vi "Initialize.vi"(8 "error in (no error)":errorcluster, 10 "DeviceName":string, 11 "FakePressureController in":refnum<class "MagAnalysis_Online.lvclass">) -> (0 "error out":errorcluster, 1 "new command(s)":string, 2 "DeviceName":string, 3 "FakePressureController out":refnum<class "MagAnalysis_Online.lvclass">)   [LabVIEW 2013, in "MagAnalysis_Online.lvclass"]
uses:
  MagAnalysis_Online.lvclass
  settings_TypDef.ctl
  CamSettings_Typdef.ctl
  CamSettingSUB_TypDEf.ctl
  MagAnalysis_Online_Bella/SubVis/CamAndObj_TypDEf.ctl
  shared/OnOffTypeDef.ctl
  SubVis/userROI.ctl
  shared/numericVariable_TypeDef.ctl
  SubVis/CamRoiTypDef.ctl
  SrewMaster_TYpDef.ctl
  srew_TypDEf.ctl
  ScrewSub_Typdef.ctl
  SubVis/screwstart.ctl
  calib_Sub_Typdef.ctl
  SubVis/ScreenCam2_TypDEf.ctl
  SubVis/ROIInfo_TypDef.ctl
  SubVis/calibPixel.ctl
  SubVis/2DTypDef.ctl
  SubVis/finalCalibTypdef.ctl
  SubVis/deltaE_FGV_typdef.ctl
  <vilib>/userdefined/High Color/IMAQdx.ctl
  BaseDriver/BaseDriver.lvclass
  MagAnalysis_Online.lvclass/MagAnalysis_Online.ctl
  SubVis/classicROI_typDef.ctl
  shared/CompressAndUpdate(Poly)/CompressAndUpdate(Numeric).vi
  <vilib>/vision/driver/NI_Vision_Acquisition_Software.lvlib
  <resource>/objmgr/imaqdx.rc
panel:
  out "Clibration.cam 0":T1={"incident ANGLE COMPENSATION"=[], "dp/B [MeV/C/B]"=[], "charge compensation"=[], "Momentum [MeV/C]"=[], "energyDependence Input"=[], "pixel angle (y)"=[], "dp [MeV/C/] "=[], "angle 2Dfor spectrumj"=[], "dp [MeV/C] 2D"=[], "charge compensation 2D"=[], "Screen&Camera 2"={"Screen Orientation"="Regular", "Screen angle"="Flat", "Lens"=enum."FL1-f8x08", "Calibration (mm/pix)"=1.0}, "ROI info"={"npix-X"=0, "npix-Y"=0, "Left [pix]"=0.0, "Top [pix]"=0.0}, "Y 2D full angle"=[], "calib pixel"={"y1(pixel)"=[], "y2(pixel)"=[], "dp/B [MeV/C/B] (pixel)"=[], "energyDependence Input(pixel)"=[], "bending angle [deg](pixel)"=[], "total path(pixel)"=[], "pixel angle (y)(pixel)"=[], "energy dependence (pixel)"=[], "charge compensation (pixel)"=[], "Momentum [MeV/C](pixel)"=[], "angular compensation(pixel)"=[]}, "2D"={"dp"=[], "chargeCompensation"=[], "angle"=[], "Momentum"=[]}, "UserROI"={"Width"=0.0, "Hight"=0.0, "OffsetX"=0.0, "OffsetY"=0.0}, "final"={"X"=[], "xi"=[], "delta momentum"=0.0, "Y"=[], "yi"=[], "angle (Y)"=[], "delta angle"=0.0, "scale delta angle"=0.0, "intraX"=0.0, "intraY"=0.0, "mask"=[]}, "B[T]"=0.0, "index"=0.0}
  out "ROI":i32[][](array[numeric])
  out "data":T9={"CamSettings"={"Cam 0"={"position"=0.0, "pixelsize"=0.0, "start"=0.0, "end"=0.0, "center"=0.0, "Lens"=enum."FL1-f8x08", "Forward"=enum."off", "Spec_Calib_file 2"=path "Y:/100TWdata/ESMCalib/datFwd.txt", "map"=path "Y:/100TWdata/ESMCalib/mapFwd.txt", "y size"=0, "UserROI"={"Width"={"Value"=0.0, "Min"=0.0, "Max"=0.0, "StepSize"=0.0, "Tolerance"=0.0, "ValueActual"=0.0}, "Hight"={"Value"=0.0, "Min"=0.0, "Max"=0.0, "StepSize"=0.0, "Tolerance"=0.0, "ValueActual"=0.0}, "OffsetX"={"Value"=0.0, "Min"=0.0, "Max"=0.0, "StepSize"=0.0, "Tolerance"=0.0, "ValueActual"=0.0}, "OffsetY"={"Value"=0.0, "Min"=0.0, "Max"=0.0, "StepSize"=0.0, "Tolerance"=0.0, "ValueActual"=0.0}}, "CamMaxPixel"={"X"=0, "Y"=0}, "CamROI"={"Width"=0.0, "Hight"=0.0, "OffsetX"=0.0, "OffsetY"=0.0}}, "Cam 1"={"position"=0.0, "pixelsize"=0.0, "start"=0.0, "end"=0.0, "center"=0.0, "Lens"=enum."FL1-f8x08", "Forward"=enum."off", "Spec_Calib_file 2"=path "Y:/100TWdata/ESMCalib/datFwd.txt", "map"=path "Y:/100TWdata/ESMCalib/mapFwd.txt", "y size"=0, "UserROI"={"Width"={"Value"=0.0, "Min"=0.0, "Max"=0.0, "StepSize"=0.0, "Tolerance"=0.0, "ValueActual"=0.0}, "Hight"={"Value"=0.0, "Min"=0.0, "Max"=0.0, "StepSize"=0.0, "Tolerance"=0.0, "ValueActual"=0.0}, "OffsetX"={"Value"=0.0, "Min"=0.0, "Max"=0.0, "StepSize"=0.0, "Tolerance"=0.0, "ValueActual"=0.0}, "OffsetY"={"Value"=0.0, "Min"=0.0, "Max"=0.0, "StepSize"=0.0, "Tolerance"=0.0, "ValueActual"=0.0}}, "CamMaxPixel"={"X"=0, "Y"=0}, "CamROI"={"Width"=0.0, "Hight"=0.0, "OffsetX"=0.0, "OffsetY"=0.0}}, "Cam 2"={"position"=0.0, "pixelsize"=0.0, "start"=0.0, "end"=0.0, "center"=0.0, "Lens"=enum."FL1-f8x08", "Forward"=enum."off", "Spec_Calib_file 2"=path "Y:/100TWdata/ESMCalib/datFwd.txt", "map"=path "Y:/100TWdata/ESMCalib/mapFwd.txt", "y size"=0, "UserROI"={"Width"={"Value"=0.0, "Min"=0.0, "Max"=0.0, "StepSize"=0.0, "Tolerance"=0.0, "ValueActual"=0.0}, "Hight"={"Value"=0.0, "Min"=0.0, "Max"=0.0, "StepSize"=0.0, "Tolerance"=0.0, "ValueActual"=0.0}, "OffsetX"={"Value"=0.0, "Min"=0.0, "Max"=0.0, "StepSize"=0.0, "Tolerance"=0.0, "ValueActual"=0.0}, "OffsetY"={"Value"=0.0, "Min"=0.0, "Max"=0.0, "StepSize"=0.0, "Tolerance"=0.0, "ValueActual"=0.0}}, "CamMaxPixel"={"X"=0, "Y"=0}, "CamROI"={"Width"=0.0, "Hight"=0.0, "OffsetX"=0.0, "OffsetY"=0.0}}, "Cam 3"={"position"=0.0, "pixelsize"=0.0, "start"=0.0, "end"=0.0, "center"=0.0, "Lens"=enum."FL1-f8x08", "Forward"=enum."off", "Spec_Calib_file 2"=path "Y:/100TWdata/ESMCalib/datFwd.txt", "map"=path "Y:/100TWdata/ESMCalib/mapFwd.txt", "y size"=0, "UserROI"={"Width"={"Value"=0.0, "Min"=0.0, "Max"=0.0, "StepSize"=0.0, "Tolerance"=0.0, "ValueActual"=0.0}, "Hight"={"Value"=0.0, "Min"=0.0, "Max"=0.0, "StepSize"=0.0, "Tolerance"=0.0, "ValueActual"=0.0}, "OffsetX"={"Value"=0.0, "Min"=0.0, "Max"=0.0, "StepSize"=0.0, "Tolerance"=0.0, "ValueActual"=0.0}, "OffsetY"={"Value"=0.0, "Min"=0.0, "Max"=0.0, "StepSize"=0.0, "Tolerance"=0.0, "ValueActual"=0.0}}, "CamMaxPixel"={"X"=0, "Y"=0}, "CamROI"={"Width"=0.0, "Hight"=0.0, "OffsetX"=0.0, "OffsetY"=0.0}}}, "timeout"={"Value"=0.0, "Min"=0.0, "Max"=0.0, "StepSize"=0.0, "Tolerance"=0.0, "ValueActual"=0.0}, "Screws"={"Cam 0"={"S 0"={"0"=0, "1"=0, "2"=0, "3"=0}, "S 1"={"0"=0, "1"=0, "2"=0, "3"=0}, "S 2"={"0"=0, "1"=0, "2"=0, "3"=0}, "S 3"={"0"=0, "1"=0, "2"=0, "3"=0}, "S 4"={"0"=0, "1"=0, "2"=0, "3"=0}, "S 5"={"0"=0, "1"=0, "2"=0, "3"=0}}, "Cam 1"={"S 0"={"0"=0, "1"=0, "2"=0, "3"=0}, "S 1"={"0"=0, "1"=0, "2"=0, "3"=0}, "S 2"={"0"=0, "1"=0, "2"=0, "3"=0}, "S 3"={"0"=0, "1"=0, "2"=0, "3"=0}, "S 4"={"0"=0, "1"=0, "2"=0, "3"=0}, "S 5"={"0"=0, "1"=0, "2"=0, "3"=0}}, "Cam 2"={"S 0"={"0"=0, "1"=0, "2"=0, "3"=0}, "S 1"={"0"=0, "1"=0, "2"=0, "3"=0}, "S 2"={"0"=0, "1"=0, "2"=0, "3"=0}, "S 3"={"0"=0, "1"=0, "2"=0, "3"=0}, "S 4"={"0"=0, "1"=0, "2"=0, "3"=0}, "S 5"={"0"=0, "1"=0, "2"=0, "3"=0}}, "Cam 3"={"S 0"={"0"=0, "1"=0, "2"=0, "3"=0}, "S 1"={"0"=0, "1"=0, "2"=0, "3"=0}, "S 2"={"0"=0, "1"=0, "2"=0, "3"=0}, "S 3"={"0"=0, "1"=0, "2"=0, "3"=0}, "S 4"={"0"=0, "1"=0, "2"=0, "3"=0}, "S 5"={"0"=0, "1"=0, "2"=0, "3"=0}}}, "number of cam"=0.0, "X size"=0.0, "srewstart"={"Cam 0"=0.0, "Cam 1"=0.0, "Cam 2"=0.0, "Cam 3"=0.0}, "Save"=enum."off", "offset"=0.0, "localsavingpath"=path "", "ROIString"="", "exposure"={"Value"=0.0, "Min"=0.0, "Max"=0.0, "StepSize"=0.0, "Tolerance"=0.0, "ValueActual"=0.0}, "trigger"=enum."off"}
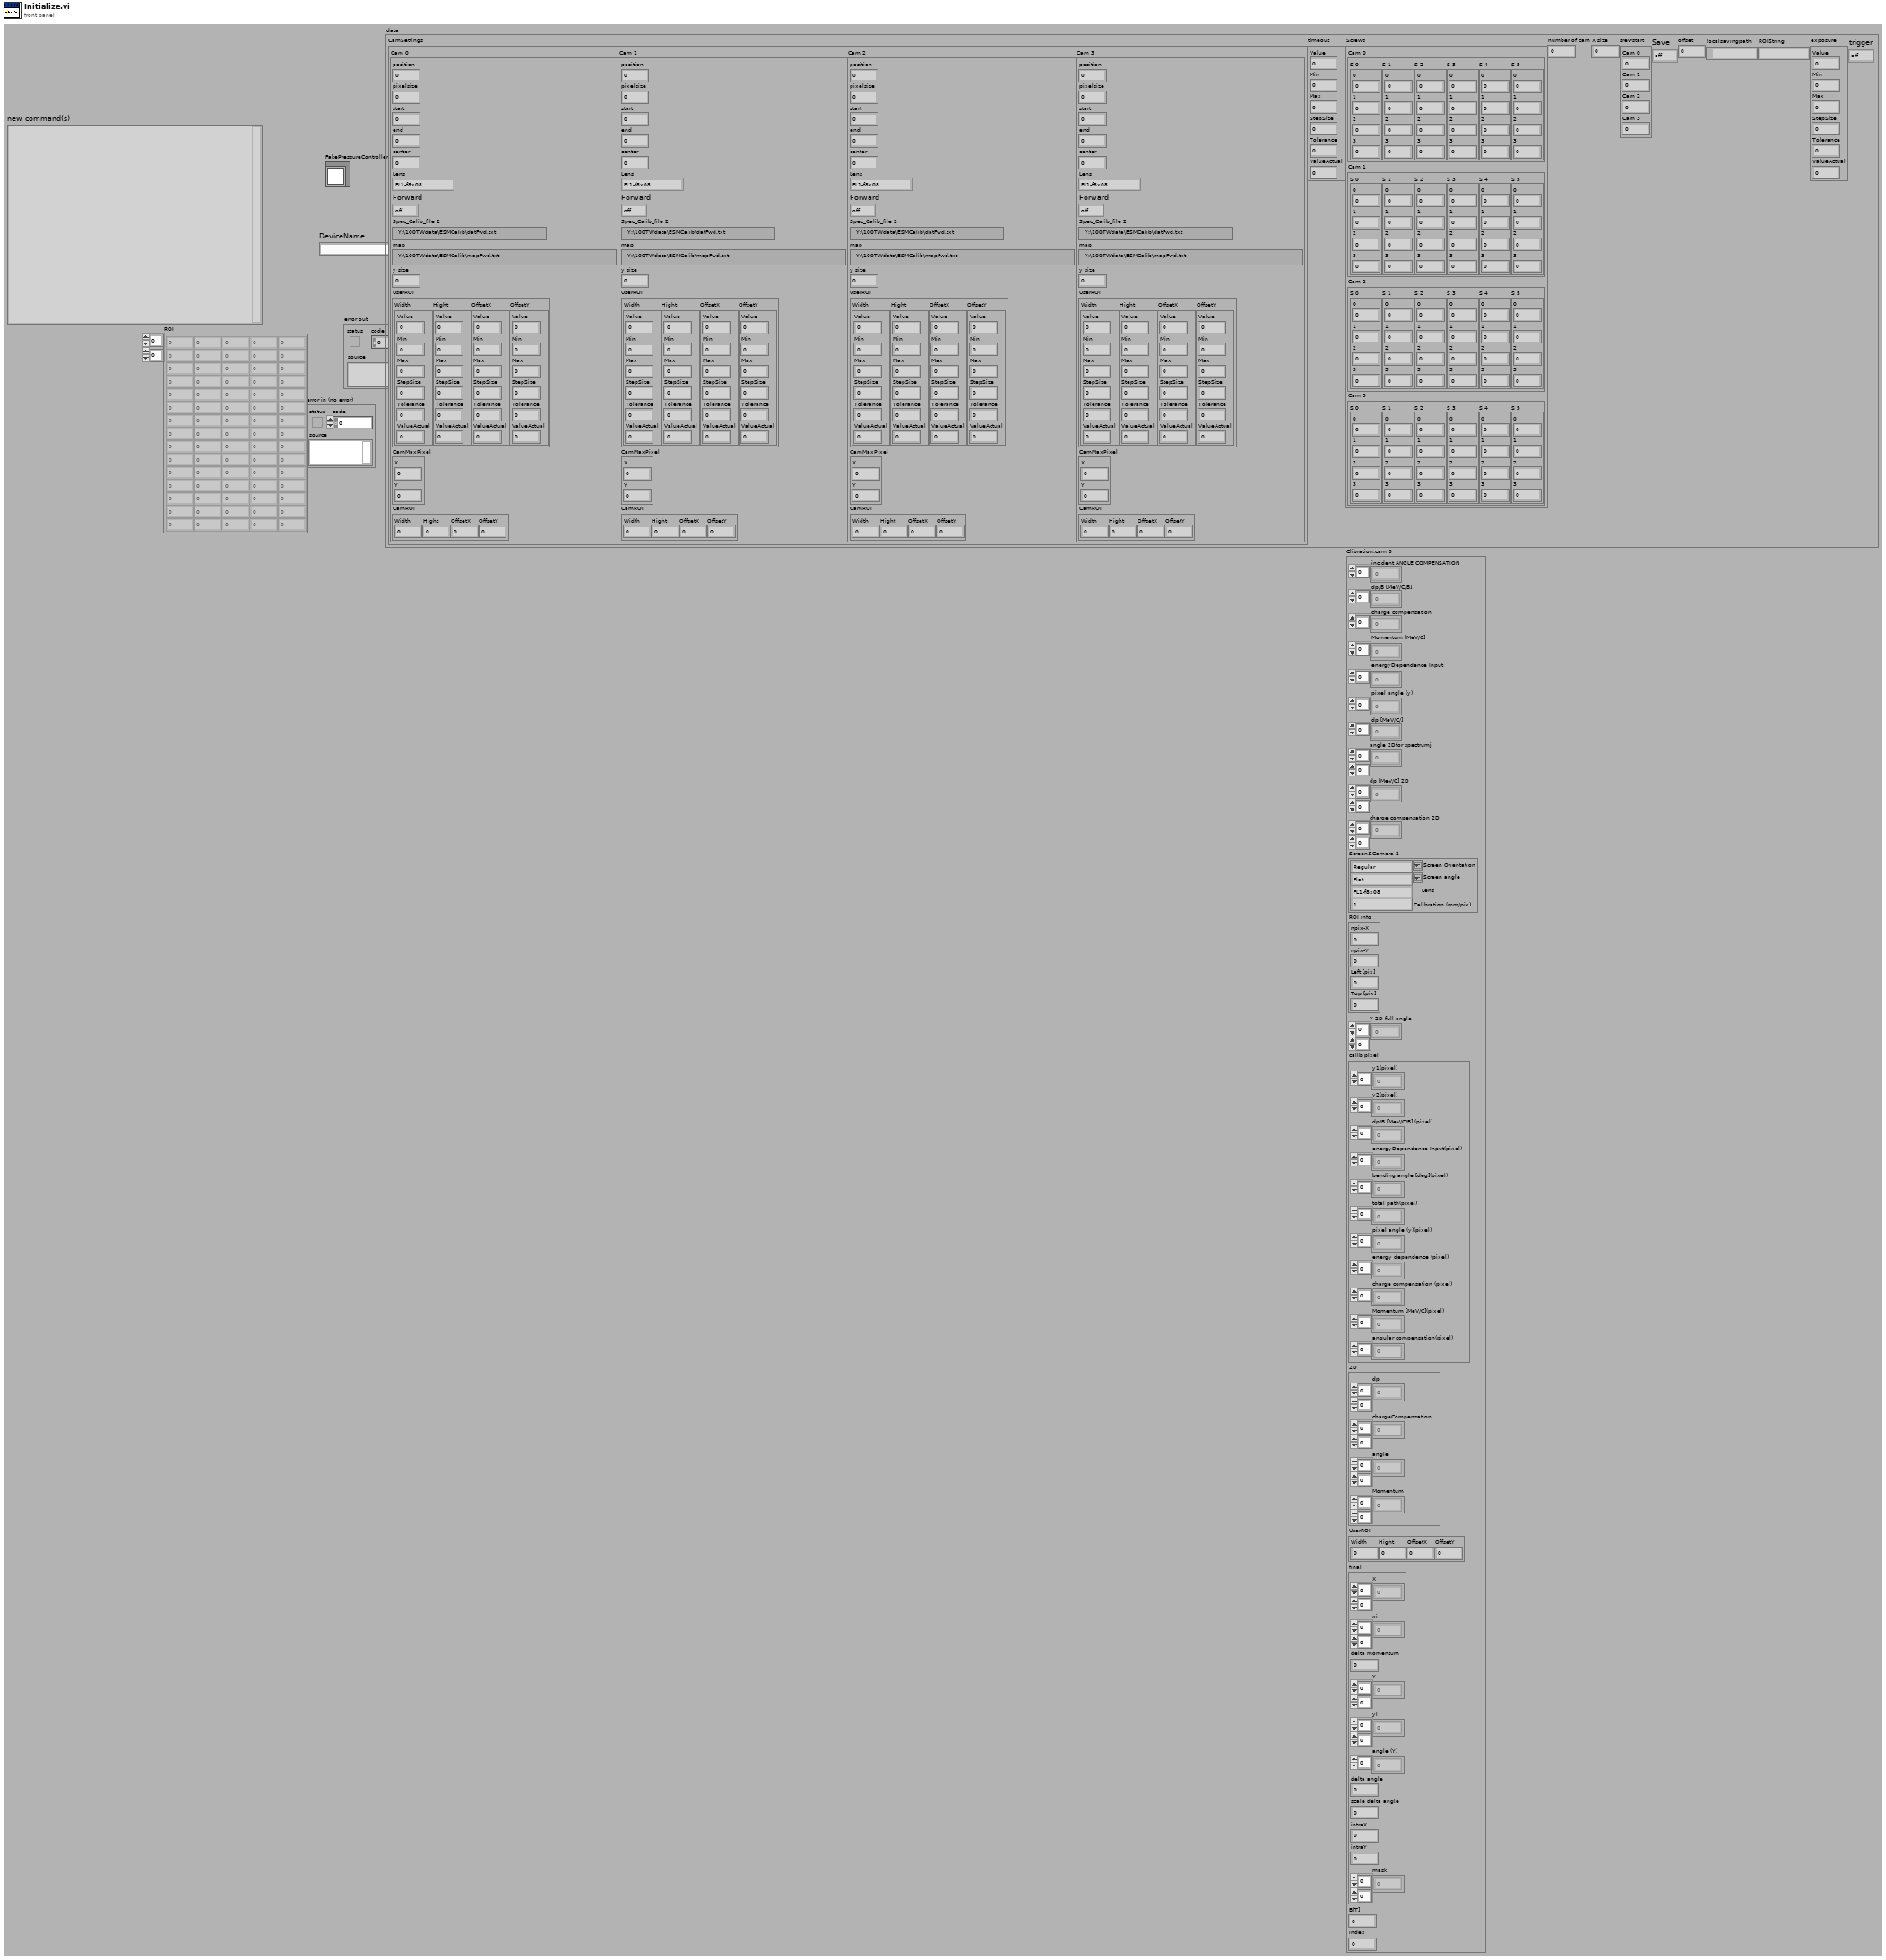
[diagram p1: front panel]
types:
  T1 = typedef "calib_Sub_Typdef.ctl" = cluster{"incident ANGLE COMPENSATION":dbl[], "dp/B [MeV/C/B]":dbl[], "charge compensation":dbl[], "Momentum [MeV/C]":dbl[], "energyDependence Input":dbl[], "pixel angle (y)":dbl[], "dp [MeV/C/] ":dbl[], "angle 2Dfor spectrumj":dbl[][], "dp [MeV/C] 2D":dbl[][], "charge compensation 2D":dbl[][], "Screen&Camera 2":T2, "ROI info":T4, "Y 2D full angle":dbl[][], "calib pixel":T5, "2D":T6, "UserROI":T7, "final":T8, "B[T]":dbl, "index":dbl}
  T2 = typedef "ScreenCam2_TypDEf.ctl" = cluster{"Screen Orientation":string, "Screen angle":string, "Lens":T3, "Calibration (mm/pix)":dbl}
  T3 = typedef "CamAndObj_TypDEf.ctl" = enum16{"FL1-f8x08", "FL1-f8x06", "FL1-f8", "ch300-f50", "FL2G-f8", "FL3M14-f8", "FL3M14-f8x08", "FL3M14-f8x08(2x2)"}
  T4 = typedef "ROIInfo_TypDef.ctl" = cluster{"npix-X":i32, "npix-Y":i32, "Left [pix]":dbl, "Top [pix]":dbl}
  T5 = typedef "calibPixel.ctl" = cluster{"y1(pixel)":dbl[], "y2(pixel)":dbl[], "dp/B [MeV/C/B] (pixel)":dbl[], "energyDependence Input(pixel)":dbl[], "bending angle [deg](pixel)":dbl[], "total path(pixel)":dbl[], "pixel angle (y)(pixel)":dbl[], "energy dependence (pixel)":dbl[], "charge compensation (pixel)":dbl[], "Momentum [MeV/C](pixel)":dbl[], "angular compensation(pixel)":dbl[]}
  T6 = typedef "2DTypDef.ctl" = cluster{"dp":dbl[][], "chargeCompensation":dbl[][], "angle":dbl[][], "Momentum":dbl[][]}
  T7 = typedef "CamRoiTypDef.ctl" = cluster{"Width":dbl, "Hight":dbl, "OffsetX":dbl, "OffsetY":dbl}
  T8 = typedef "finalCalibTypdef.ctl" = cluster{"X":dbl[][], "xi":dbl[][], "delta momentum":dbl, "Y":dbl[][], "yi":dbl[][], "angle (Y)":dbl[], "delta angle":dbl, "scale delta angle":dbl, "intraX":dbl, "intraY":dbl, "mask":dbl[][]}
  T9 = typedef "MagAnalysis_Online.lvclass/settings_TypDef.ctl" = cluster{"CamSettings":T10, "timeout":T14, "Screws":T15, "number of cam":dbl, "X size":dbl, "srewstart":T18, "Save":T12, "offset":dbl, "localsavingpath":path, "ROIString":string, "exposure":T14, "trigger":T12}
  T10 = typedef "CamSettings_Typdef.ctl" = cluster{"Cam 0":T11, "Cam 1":T11, "Cam 2":T11, "Cam 3":T11}
  T11 = typedef "CamSettingSUB_TypDEf.ctl" = cluster{"position":dbl, "pixelsize":dbl, "start":dbl, "end":dbl, "center":dbl, "Lens":T3, "Forward":T12, "Spec_Calib_file 2":path, "map":path, "y size":i32, "UserROI":T13, "CamMaxPixel":cluster{"X":i32, "Y":i32}, "CamROI":T7}
  T12 = typedef "OnOffTypeDef.ctl" = enum16{"off", "on"}
  T13 = typedef "userROI.ctl" = cluster{"Width":T14, "Hight":T14, "OffsetX":T14, "OffsetY":T14}
  T14 = typedef "BaseDriver.lvclass/numericVariable_TypeDef.ctl" = cluster{"Value":dbl, "Min":dbl, "Max":dbl, "StepSize":dbl, "Tolerance":dbl, "ValueActual":dbl}
  T15 = typedef "SrewMaster_TYpDef.ctl" = cluster{"Cam 0":T16, "Cam 1":T16, "Cam 2":T16, "Cam 3":T16}
  T16 = typedef "srew_TypDEf.ctl" = cluster{"S 0":T17, "S 1":T17, "S 2":T17, "S 3":T17, "S 4":T17, "S 5":T17}
  T17 = typedef "ScrewSub_Typdef.ctl" = cluster{"0":i32, "1":i32, "2":i32, "3":i32}
  T18 = typedef "screwstart.ctl" = cluster{"Cam 0":dbl, "Cam 1":dbl, "Cam 2":dbl, "Cam 3":dbl}
  T19 = typedef "IMAQdx.ctl" = refnum<k21>
  T20 = typedef "deltaE_FGV_typdef.ctl" = enum16{"init", "set", "read"}
  T21 = typedef "Image Type" = u32
  T22 = typedef "IMAQ Image.ctl" = refnum<image>
  T23 = typedef "MagAnalysis_Online.lvclass/analysis_data_typdef.ctl" = cluster{"cam0":T22, "cam1":T22, "cam2":T22, "cam3":T22}
  T24 = typedef "bgImages_tyudef.ctl" = cluster{"cam 0":T22, "cam 1":T22, "cam 2":T22, "cam 3":T22}
  T25 = typedef "configTypDEf.ctl" = cluster{"bending angle":dbl[], "screen [m]":dbl[], "momentum [MeV/c]":dbl[], "total path [m]":dbl[], "x[mm](rms)":dbl[], "x[mm](rms,b)":dbl[], "y[mm](rms)":dbl[], "y[mm](rms,b)":dbl[]}
  T26 = cluster{"[0]":T25, "[1]":T25, "[2]":T25, "[3]":T25}
  T27 = typedef "classicROI_typDef.ctl" = cluster{"Width":dbl, "Hight":dbl, "OffsetX":dbl, "OffsetY":dbl}
  T28 = cluster{"[0]":T27, "[1]":T27, "[2]":T27, "[3]":T27}
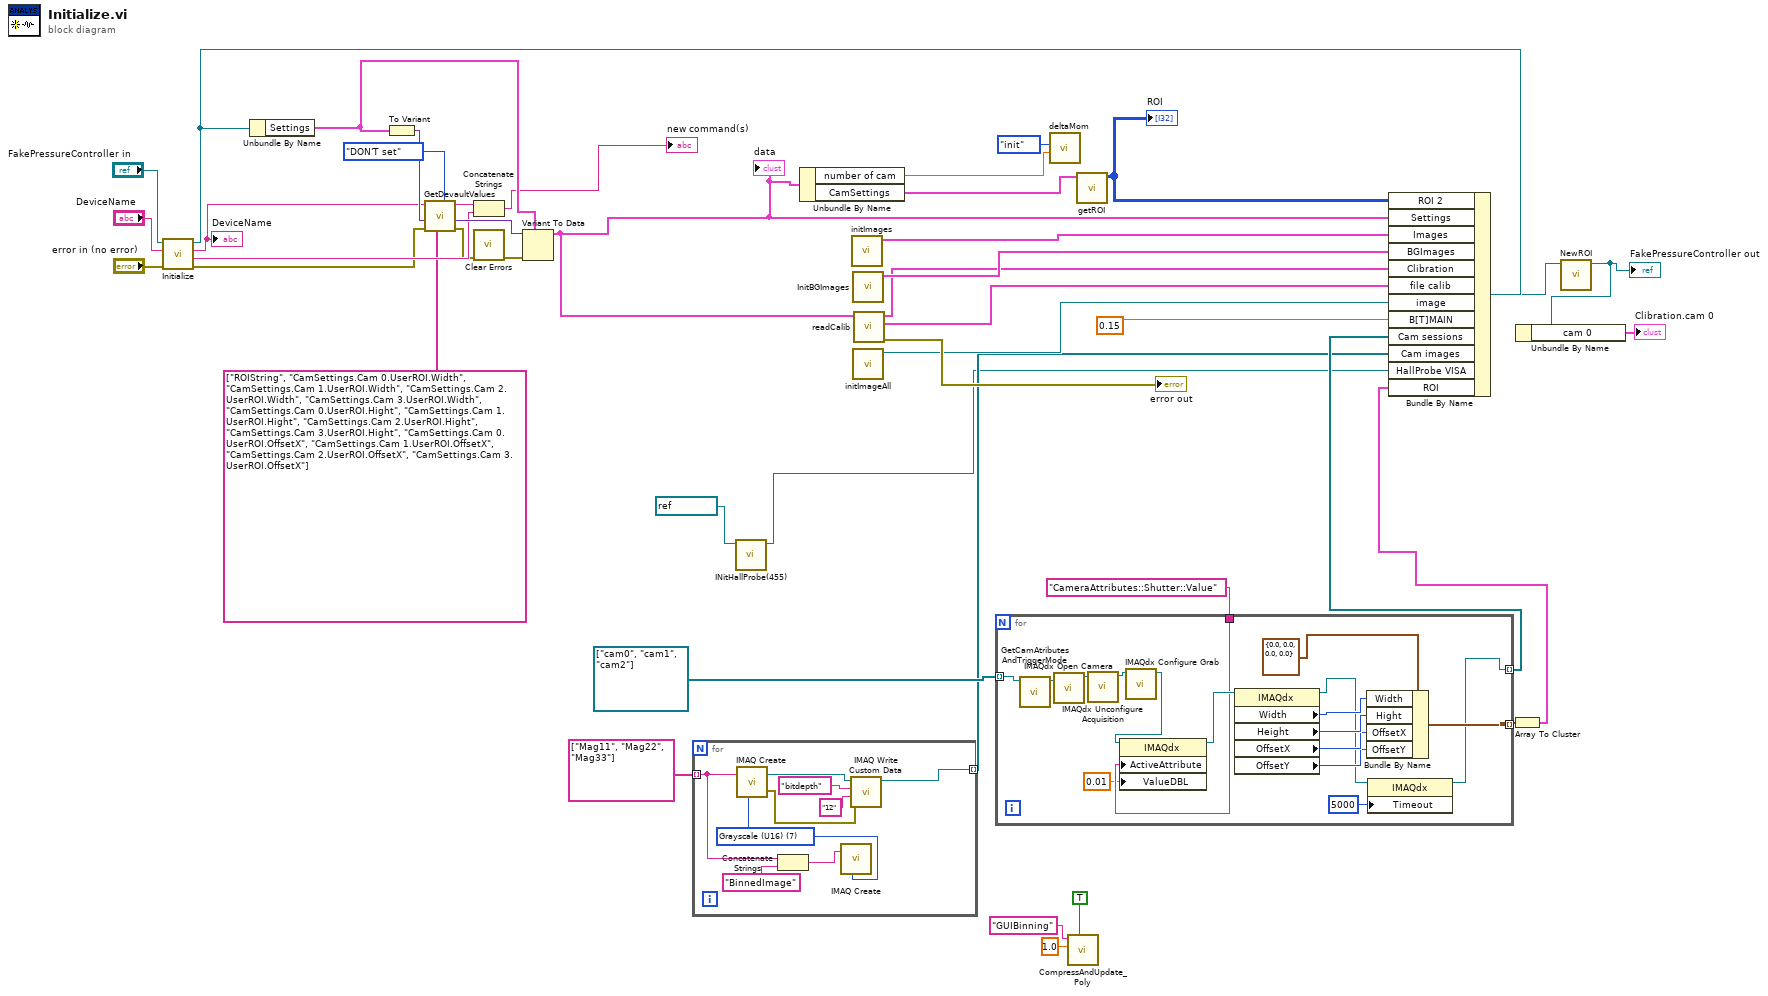
[diagram p0: block diagram]
diagram:
  n1 = call-parent "Initialize.vi"("error in (no error)"="error in (no error)", "DeviceName"="DeviceName", "BaseDriver in"="FakePressureController in") -> ("error out"=w35:errorcluster, "new command(s)"=w36:string, "DeviceName"=w34:string, "BaseDriver out"=w28:refnum<class "MagAnalysis_Online.lvclass">)  [unwired: 5 in]
  "DeviceName" <- w34
  n2 = Unbundle By Name(w28) -> ("Settings"=w37:T9)
  n3 = To Variant(anything=w37) -> (Variant=w38:variant)
  n4 = call "GetDevaultValues.vi"("set or DON'T set"=enum16{"set", "DON'T set"}."DON'T set", "set following Variables (empty = all avriables)"=string[] ["ROIString", "CamSettings.Cam 0.UserROI.Width", "CamSettings.Cam 1.UserROI.Width", "CamSettings.Cam 2.UserROI.Width", "CamSettings.Cam 3.UserROI.Width", "CamSettings.Cam 0.UserROI.Hight", "CamSettings.Cam 1.UserROI.Hight", "CamSettings.Cam 2.UserROI.Hight", "CamSettings.Cam 3.UserROI.Hight", "CamSettings.Cam 0.UserROI.OffsetX", "CamSettings.Cam 1.UserROI.OffsetX", "CamSettings.Cam 2.UserROI.OffsetX", "CamSettings.Cam 3.UserROI.OffsetX"], "error in (no error)"=w35, "variant"=w38, "Device Name"=w34) -> ("error out"=w33:errorcluster, "variant out"=w39:variant, "new command(s)"=w40:string)  [unwired: 4 in]
  n5 = Concatenate Strings(w40, w36) -> (→"new command(s)":string)
  n6 = call <vilib>:"Clear Errors.vi"("error in (no error)"=w33) -> ("error out"=w32:errorcluster)  [unwired: 6 in]
  n7 = Variant To Data(error in=w32, type=w37, Variant=w39) -> (data=w17:T9)  [unwired: 1 out]
  "data" <- w17
  n8 = for {
    tunnel: string[] ["Mag11", "Mag22", "Mag33"] -> [w51] mode=indexing
    tunnel: [w48] -> w11 mode=indexing
    w44 = T21 7 items=["Grayscale (U8)", "Grayscale (I16)", "Grayscale (SGL)", "Complex (CSG)", "RGB (U32)", "HSL (U32)", "RGB (U64)", "Grayscale (U16)"] ("Image Type")
    n9 = call "IMAQ Create"("Image Name"=w51, "Image Type"=w44) -> ("New Image"=w49:T22, "error out"=w47:errorcluster)  [unwired: 3 in]
    n10 = Concatenate Strings(w51, "BinnedImage" ("command or variable name")) -> (w50:string)
    n11 = call "IMAQ Create"("Image Name"=w50, "Image Type"=w44) -> ()  [unwired: 3 in, 2 out]
    n12 = call "IMAQ Write Custom Data"("error in (no error)"=w47, "Custom Data In"="12", "Key"="bitdepth", "Image"=w49) -> ("Image Out"=w48:T22)  [unwired: 6 in, 1 out]
  }
  n13 = call "INitHallProbe(455).vi"("VISA Refnum in"=refnum<visa-resource-name> "COM1") -> ("VISA Refnum out"=w10:refnum<visa-resource-name>)  [unwired: 9 in, 1 out]
  n14 = Unbundle By Name(w17) -> ("number of cam"=w21:dbl, "CamSettings"=w16:T10)
  n15 = call "initImages.vi"() -> ("output cluster"=w29:T23)  [unwired: 11 in]
  n16 = call "InitBGImages.vi"() -> ("BGImages"=w31:T24)  [unwired: 11 in]
  n17 = call "initImageAll.vi"() -> ("Refnum out"=w25:T22)  [unwired: 11 in]
  n18 = call "readCalib.vi"("Settings"=w17) -> ("error out"=→"error out":errorcluster, "fileCalib"=w24:T26, "CamCalib"=w30:cluster{"[0]":T1, "[1]":T1, "[2]":T1, "[3]":T1})  [unwired: 8 in]
  n19 = for {
    tunnel: T19[] ["cam0", "cam1", "cam2"] -> [w66] mode=indexing
    tunnel: [w54] -> w13 mode=indexing
    tunnel: [w60] -> w9 mode=indexing
    tunnel: "CameraAttributes::Shutter::Value" -> [w57]
    n20 = call "GetCamAtributesAndTriggerMode.vi"("IMAQdx Session"=w66) -> ("IMAQdx Session 2"=w69:T19)  [unwired: 6 in, 4 out]
    n21 = call <vilib>:"IMAQdx Open Camera.vi"("Session In"=w69) -> ("Session Out"=w68:T19)  [unwired: 2 in, 8 out]
    n22 = call <vilib>:"IMAQdx Unconfigure Acquisition.vi"("Session In"=w68) -> ("Session Out"=w67:T19)  [unwired: 1 in, 9 out]
    n23 = call <vilib>:"IMAQdx Configure Grab.vi"("Session In"=w67) -> ("Session Out"=w59:T19)  [unwired: 1 in, 9 out]
    n24 = property class="IMAQdx"(reference=w59, "ActiveAttribute"=w57, "ValueDBL"=0.01) -> (reference out=w58:T19)  [unwired: 1 in, 1 out]
    n25 = property class="IMAQdx"(reference=w58) -> (reference out=w55:T19, "Width"=w64:u32, "Height"=w63:u32, "OffsetX"=w62:u32, "OffsetY"=w61:u32)  [unwired: 1 in, 1 out]
    n26 = Bundle By Name(cluster=T27 {"Width"=0.0, "Hight"=0.0, "OffsetX"=0.0, "OffsetY"=0.0} ("Cam3"), "Width"=w64, "Hight"=w63, "OffsetX"=w62, "OffsetY"=w61) -> (w60:T27)
    n27 = property class="IMAQdx"(reference=w55, "Timeout"=u32 5000) -> (reference out=w54:T19)  [unwired: 1 in, 1 out]
  }
  n28 = call "deltaMom.vi"("index"=w21, "command"=deltaE_FGV_typdef."init") -> ()  [unwired: 9 in, 1 out]
  n29 = call-poly "CompressAndUpdate_Poly.vi"("force CVT update (false)"=TRUE, "Numeric"=1.0, "command or variable name"="GUIBinning") -> ()  [unwired: 8 in, 1 out]
  n30 = call "getROI.vi"("CamSettings"=w16) -> ("ROI"=w15:i32[][])  [unwired: 10 in]
  "ROI" <- w15
  n31 = Array To Cluster(array=w9) -> (cluster=w8:T28)
  n32 = Bundle By Name(cluster=w28, "ROI 2"=w15, "Settings"=w17, "Images"=w29, "BGImages"=w31, "Clibration"=w30, "file calib"=w24, "image"=w25, "B[T]MAIN"=0.15, "Cam sessions"=w13, "Cam images"=w11, "HallProbe VISA"=w10, "ROI"=w8) -> (w27:refnum<class "MagAnalysis_Online.lvclass">)
  n33 = call "NewROI.vi"("MagAnalysis_Online in"=w27) -> ("MagAnalysis_Online out"=w3:refnum<class "MagAnalysis_Online.lvclass">)  [unwired: 10 in]
  "FakePressureController out" <- w3
  n34 = Unbundle By Name(w3) -> ("cam 0"=→"Clibration.cam 0":T1)
